vi "CSM - Running Log - DebugTool.vi"() -> ()   [LabVIEW 2017]
doc: "### CSM - Running Log - DebugTool.vi\n\nReal-time tool for viewing the running log of the entire CSM program."
uses:
  _Support/Typedef/_CSM_GlobalLog_MSG.ctl
  _Support/Typedef/_CSM_Response Source Message.ctl
  _Support/Typedef/_CSM_GlobalLog_MSG_TYPE.ctl
  _Support/GlobalEvent/GEvt-Generate with Rule Check.vi
  AdvanceAPI/CSM - Convert Error to Argument.vi
  AdvanceAPI/CSM - Make String Arguments Safe.vi
  AdvanceAPI/CSM - Keywords.vi
  _Support/GlobalEvent/LogFilter/LogFilter - Check.vi
  _Support/GlobalEvent/Cache-GEvt Refs.vi
  _Support/GlobalEvent/LogFilter/LogFilter.lvclass
  Communicable State Machine.lvlib
  addons/Logger/CSM File Logger.lvlib
  _Support/csm-tool-support.lvlib
  _csmHelper/API with lvcsm Support/CSM-Helper API with lvcsm Support.lvlib
panel:
  in  "Check Periodic Messages":bool
  in  "Filter Peroid Logs":bool
  in  "Record.Stop":bool
  in  "Record.Start":bool
  in  "BackTop":bool
  in  "Toolbar.History Length(char)":i32=50000 caption="History(char)" min=1000 max=100000000 step=1
  in  "Clear":bool
  in  "CSM":string(combo)
  in  "Search Button":bool
  in  "Toolbar.Open BD":bool
  in  "Toolbar.Open FP":bool
  out "State History":string
  in  "Tab":enum32{"Error History", "Broadcast Registry"}(tab)
  out "Error History":string
  out "Broadcast Registry":string[][](table)
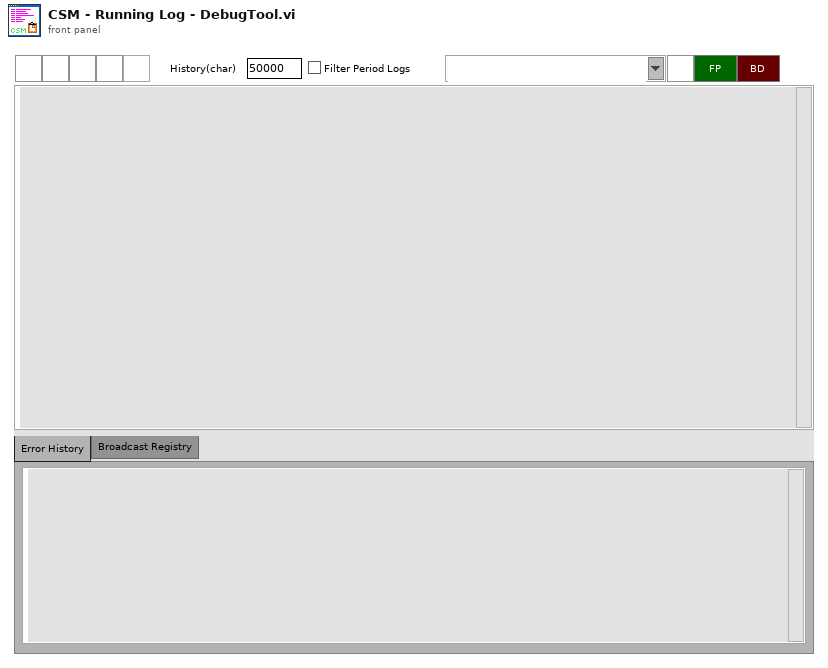
[diagram p1: front panel]
types:
  T1 = cluster{"threashold(#/s)":dbl, "Check Peroid(s)":dbl}
  T2 = typedef "Communicable State Machine.lvlib/_CSM_GlobalLog_MSG.ctl" = cluster{"Name (\"\" to Use UUID)":string, "Current State":string, "Arguments":string, "Source Message":T3, "Source Module":string, "Complete(T)/Start(F)":bool, "LogType":T4, "Time Stamp":timestamp}
  T3 = typedef "Communicable State Machine.lvlib/_CSM_Response Source Message.ctl" = cluster{"‘State":string, "’Arguments":string, "’Error":errorcluster}
  T4 = typedef "Communicable State Machine.lvlib/_CSM_GlobalLog_MSG_TYPE.ctl" = enum16{"User Log", "State Change", "Status", "Interrupt", "Register", "Unregister", "Error Log", "Module Created", "Module Destroyed", "Async Message", "No-Rep Async Message", "Sync Message"}
  T5 = enum32{"Invalid", "Standard", "Closed", "Hidden", "Minimized", "Maximized"}
  T6 = enum32{"invalid app kind", "Development System", "Run Time System", "Student Edition", "Embedded LabVIEW", "Evaluation", "Custom"}
  T7 = typedef "LVPoint32TypeDef.ctl" = cluster{"Horizontal":i32, "Vertical":i32}
  T8 = cluster{"Shift":bool, "Ctrl":bool, "Alt":bool, "Cmd":bool, "Opt":bool}
  T9 = cluster{"Core":cluster{"Current VI Reference":refnum<vi>, "Close Panel on Exit?":bool}, "Toolbar.Advance":refnum<vi>[], "LoggerWatchDogQueue":refnum<queue>, "LogFile":path}
  T10 = cluster{"Current VI Reference":refnum<vi>, "Close Panel on Exit?":bool}
  T11 = typedef "Communicable State Machine.lvlib/CSM - Broadcast Message Type.ctl" = enum16{"<Null>", "Status", "Interrupt"}
  T12 = cluster{string, "Name":string, "Target CSM":string, "Target State":string, "Register Type":T11}[]
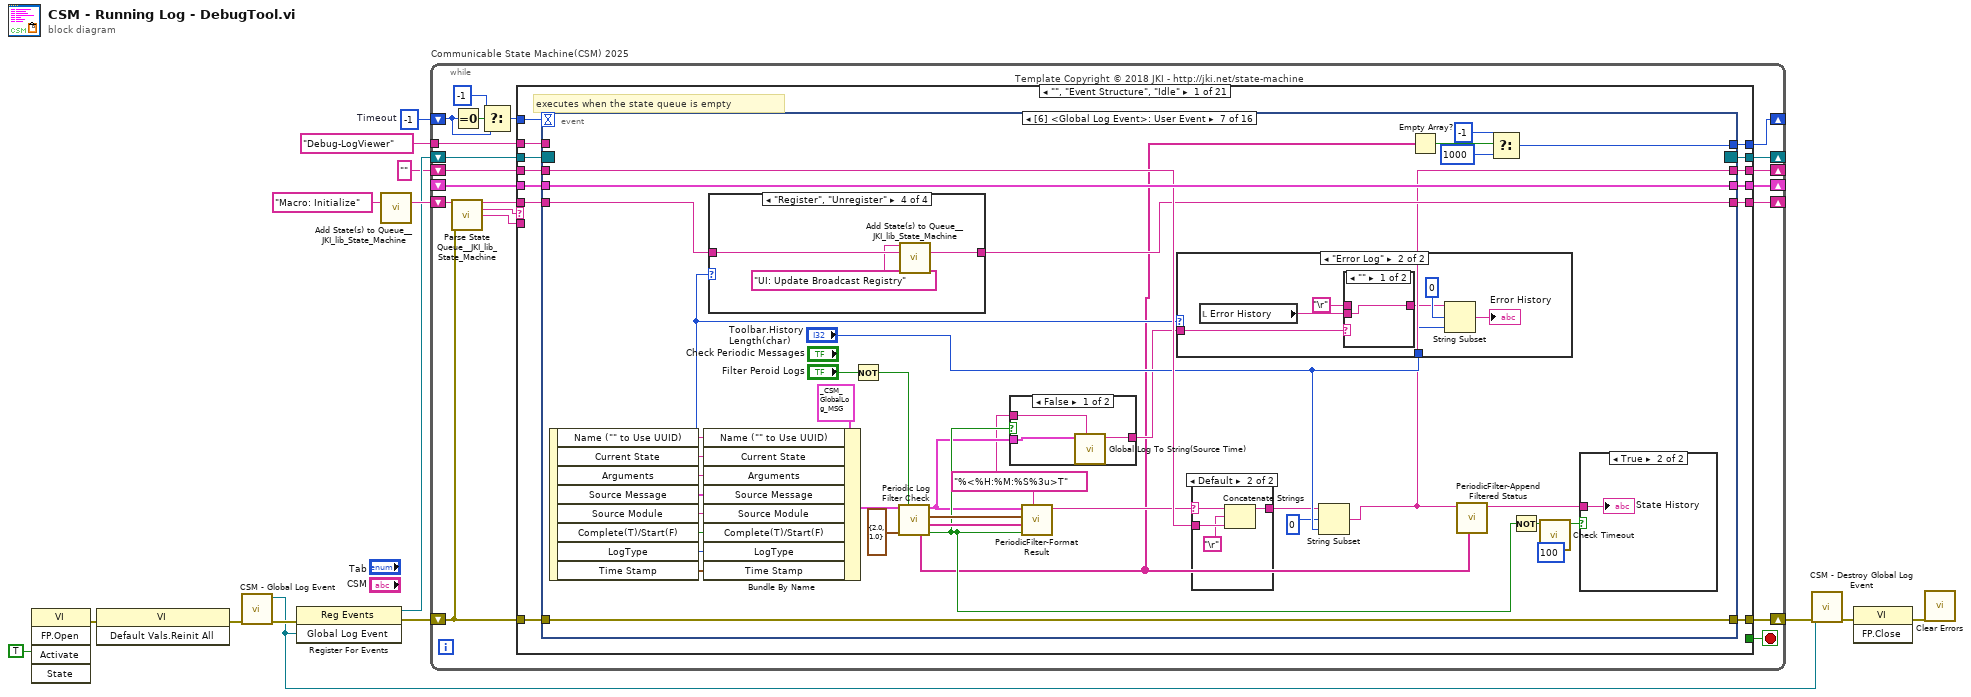
[diagram p0: block diagram]
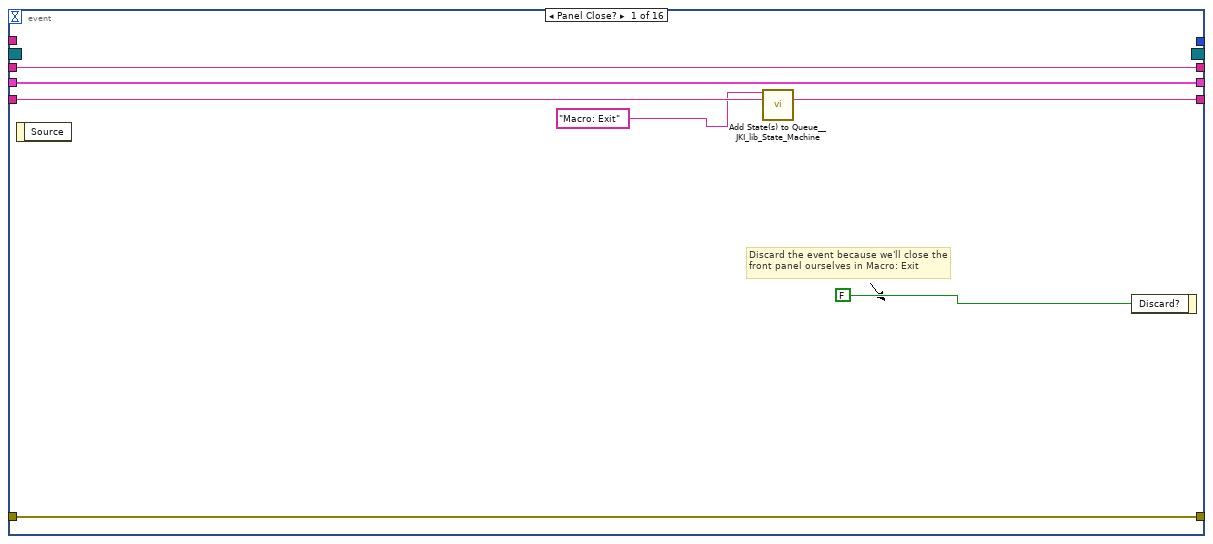
[diagram p2: hidden frame]
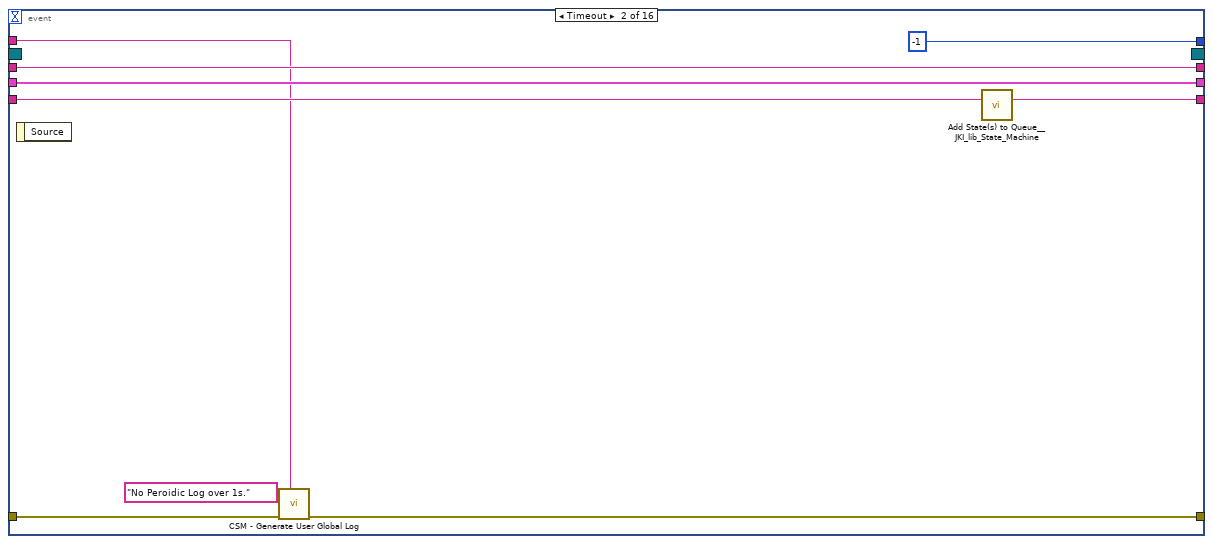
[diagram p3: hidden frame]
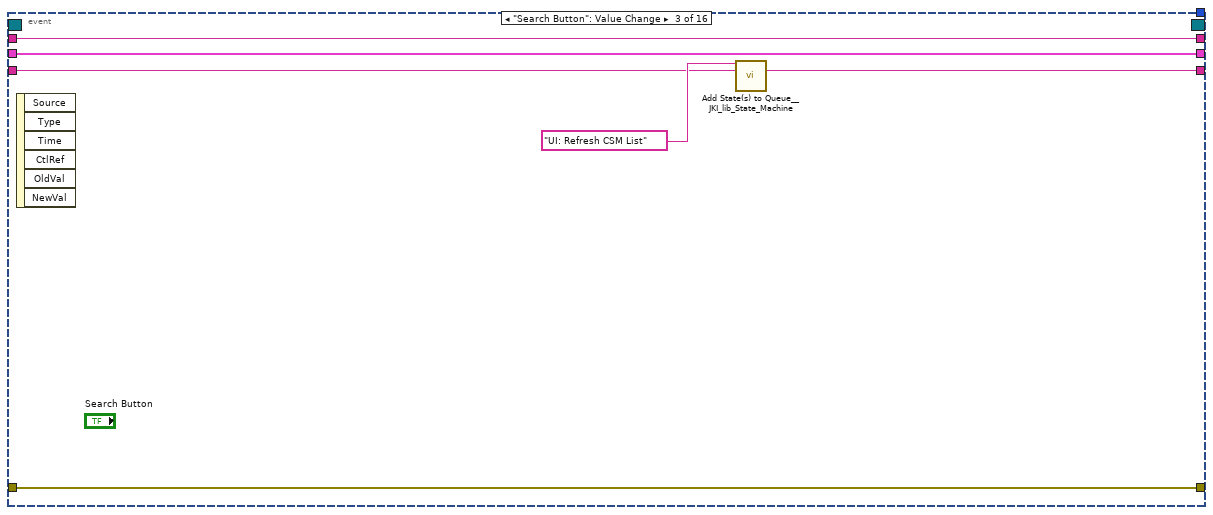
[diagram p4: hidden frame]
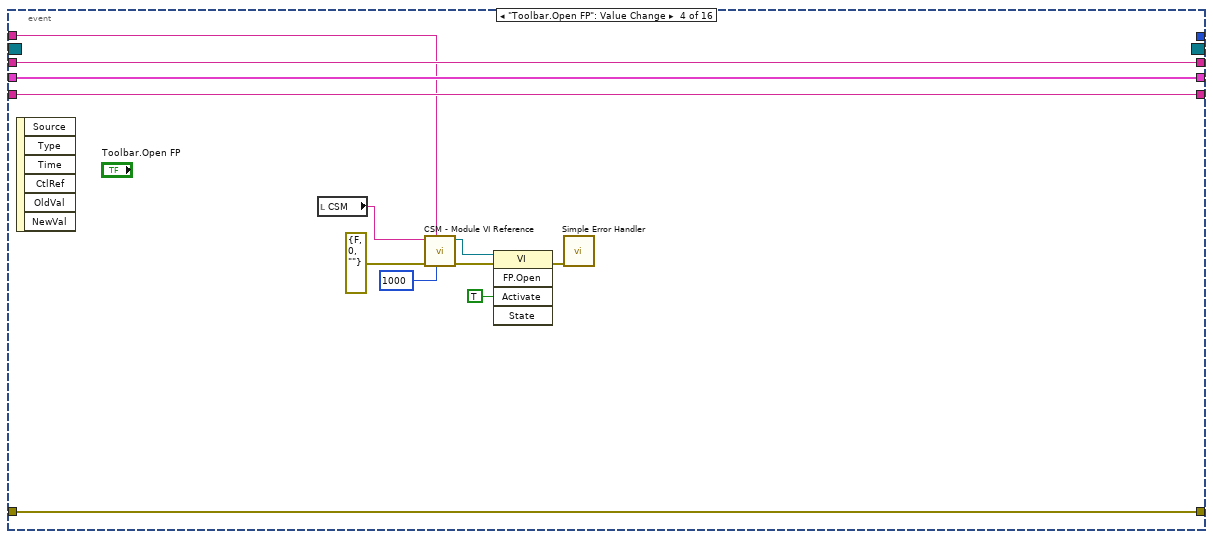
[diagram p5: hidden frame]
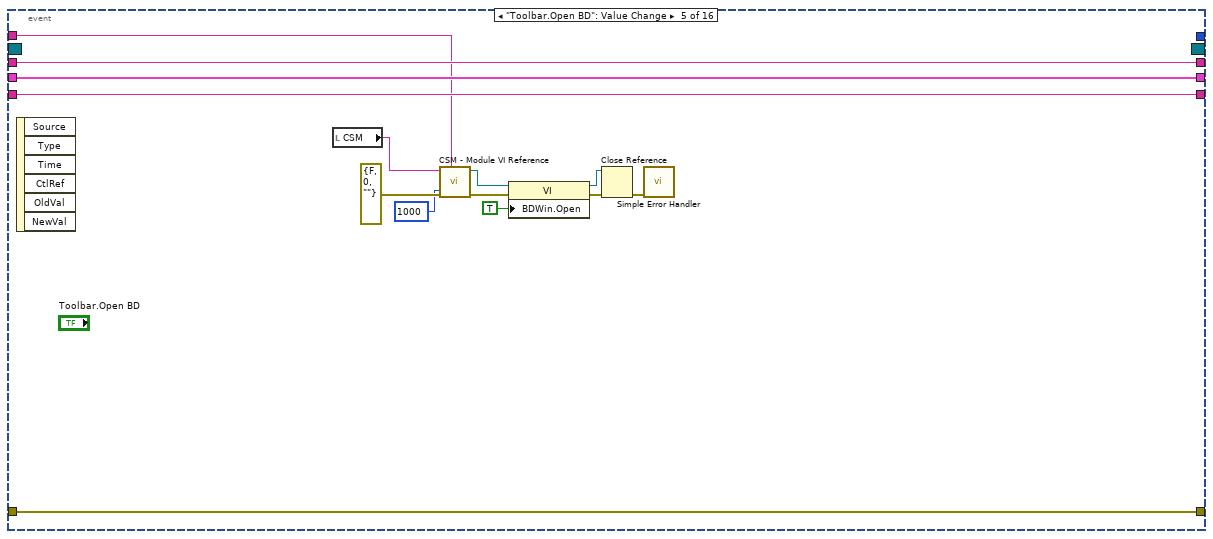
[diagram p6: hidden frame]
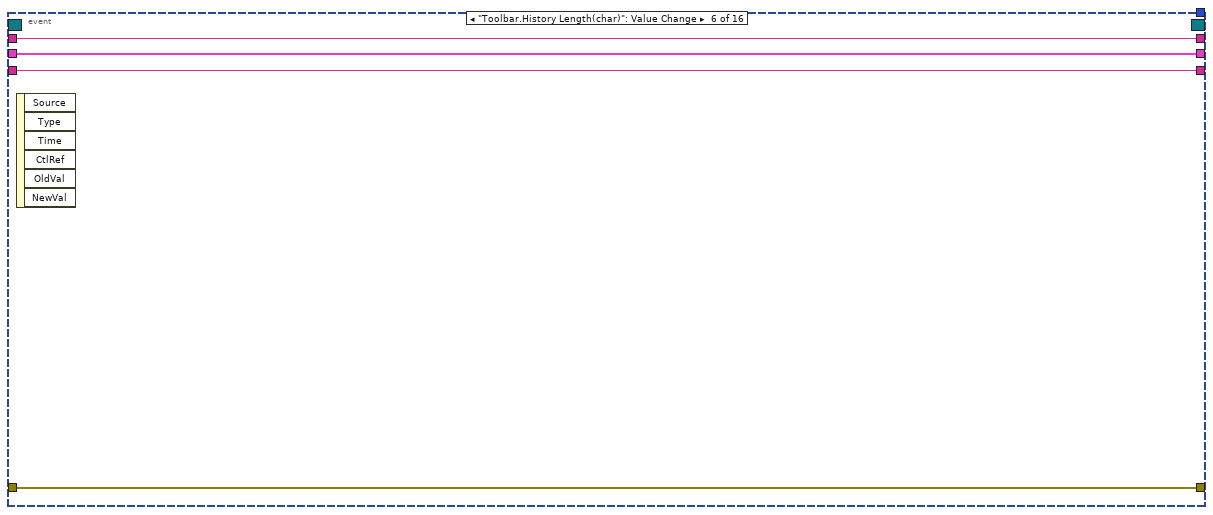
[diagram p7: hidden frame]
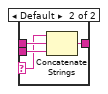
[diagram p12: hidden frame]
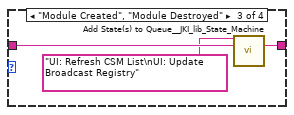
[diagram p15: hidden frame]
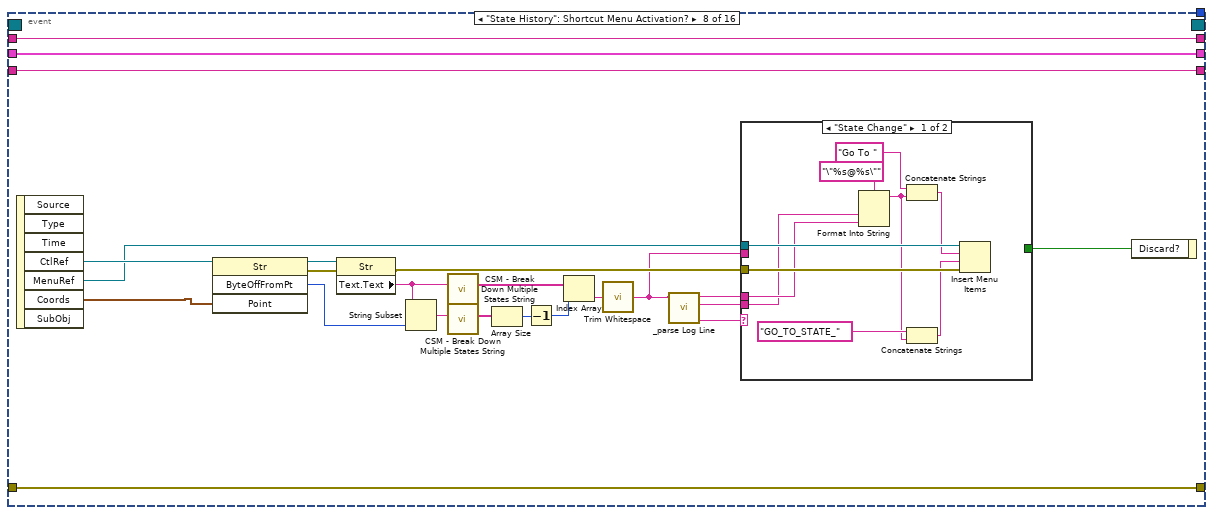
[diagram p16: hidden frame]
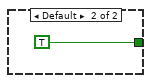
[diagram p17: hidden frame]
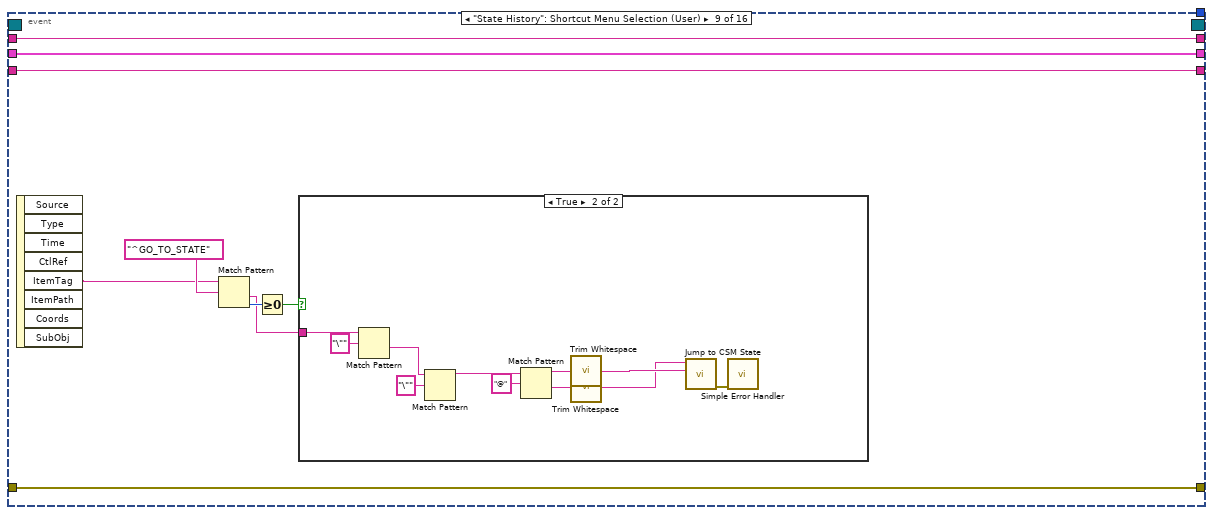
[diagram p18: hidden frame]
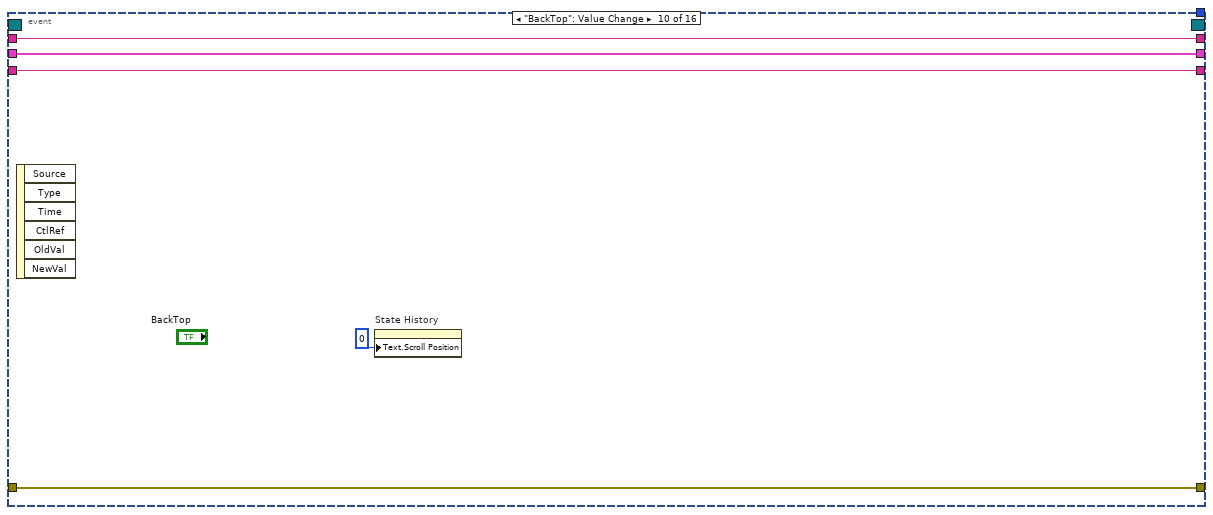
[diagram p20: hidden frame]
diagram:
  w1 = -1  # Timeout
  n1 = invoke class="VI" method="FP.Open"("Activate"=TRUE ("Activate?")) -> (error out=w14:errorcluster)  [unwired: 4 in, 4 out]
  n2 = invoke class="VI" method="Default Vals.Reinit All"(error in=w14) -> (error out=w8:errorcluster)  [unwired: 2 in, 2 out]
  n3 = call "CSM - Global Log Event.vi"("Error In"=w8) -> ("error out"=w12:errorcluster, "Global Log Event"=w11:refnum<user-event>)  [unwired: 9 in]
  n4 = register-events(error in=w12, w11) -> (reference out=w6:refnum<event-registration>, error out=w7:errorcluster)  [unwired: 1 in]
  n5 = call <vilib>:"Add State(s) to Queue__JKI_lib_State_Machine.vi"("State(s) in (\"\")"="Macro: Initialize") -> ("States Out"=w10:string)  [unwired: 14 in]
  n6 = while "Communicable State Machine(CSM) 2025" {
    shift-right: [w28] -> _
    shift-left: _ -> [w27]
    shift-right: [w31] -> w5
    shift-left: w7 -> [w26]
    shift-right: [w30] -> _
    shift-left: w10 -> [w32]
    shift-right: [w24] -> _
    shift-left: w6 -> [w25]
    tunnel: "Debug-LogViewer" ("Current Module(\"\" to generate an ID)") -> [w23]
    shift-right: [w21] -> _
    shift-left: "" ("String Cache") -> [w22]
    shift-right: [w20] -> _
    shift-left: w1 -> [w17]
    stop <- w29 stop-if-true
    # "Template Copyright © 2018 JKI - http://jki.net/state-machine"
    n7 = call <vilib>:"Parse State Queue__JKI_lib_State_Machine.vi"("State Queue"=w32, "Error In (no error)"=w26) -> ("Remaining States"=w34:string, "Current State"=w35:string, "Arguments"=w33:string)  [unwired: 11 in]
    n8 = Equal To 0?(x=w17) -> (x = 0?=w19:bool)
    n9 = Select(t=-1 ("Timeout"), s=w19, f=w17) -> (s? t:f=w18:i32)
    n10 = case shown="\"\", \"Event Structure\", \"Idle\"" w35 {
      selector: w35 -> [_ _ w296 _ _ _ _ _ _ _ _ _ _ _ _ _ _ _ _ _ _]
      tunnel: w34 -> [w48 w292 w300 w322 w331 w339 w346 w357 w367 w376 w383 w392 w404 w418 w495 w503 w532 w556 w564 w572 w585]
      tunnel: w33 -> [_ _ _ _ _ _ _ _ _ _ _ _ w399 w412 _ _ _ _ _ _ _]
      tunnel: w27 -> [w46 w289 w298 w315 w328 w337 w343 _ w366 w371 w380 w387 w402 w414 w494 w502 w527 w555 w561 w569 w582]
      tunnel: [w45 w290 w302 w319 errorcluster {"status"=FALSE, "code"=0, "source"=""} ("error out") w336 w344 w354 w359 w372 w381 w390 w400 w415 w496 w504 w533 w557 w562 w570 w583] -> w31
      tunnel: w26 -> [w44 w290 w301 w319 w327 w336 w344 w354 w359 w373 w381 w390 w401 w416 w496 w504 w533 w557 w562 w570 w583]
      tunnel: [w47 w291 w299 w321 w330 w338 w345 w356 w367 w375 w382 w391 w403 w417 w495 w503 w532 w556 w563 w571 w584] -> w30
      tunnel: [_ _ _ _ _ TRUE _ _ _ _ _ _ _ _ _ _ _ _ _ _ _] -> w29
      tunnel: [w43 w289 w298 w320 w328 w337 w343 w355 w363 w371 w380 w387 w402 w414 w494 w502 w527 w555 w561 w569 w582] -> w28
      tunnel: w18 -> [w42 w286 w293 w307 w323 w332 w340 w347 w358 w368 w377 w384 w396 w409 w484 w497 w513 w540 w558 w565 w573]
      tunnel: w25 -> [w41 w288 w295 w309 w325 w334 w342 w352 w365 w370 w379 w389 w398 w411 w493 w501 w531 w554 w560 w567 w575]
      tunnel: [w40 w288 w295 w309 w325 w334 w342 w352 w365 w370 w379 w389 w398 w411 w493 w501 w531 w554 w560 w567 w575] -> w24
      tunnel: w23 -> [w39 _ _ _ _ _ _ _ _ _ _ _ _ _ _ _ _ _ _ _ _]
      tunnel: w22 -> [w38 w287 w294 w308 w324 w333 w341 w351 w364 w369 w378 w388 w397 w410 w492 w500 w530 w553 w559 w566 w574]
      tunnel: [w37 w287 w294 w308 w324 w333 w341 w351 w364 w369 w378 w388 w397 w410 w492 w500 w530 w553 w559 w566 w574] -> w21
      tunnel: [w36 w286 w293 w307 w323 w332 w340 w347 w358 w368 w377 w384 w396 w409 w484 w497 w513 w540 w558 w565 w573] -> w20
      frame "", "Event Structure", "Idle" {
        # "executes when the state queue is empty"
        n11 = event shown="[6] <Global Log Event>: User Event" {
          selector: w41 -> [_ _ _ _ _ _ _ _ _ _ _ _ _ _ _ _]
          dyn-events: [_ _ _ _ _ _ _ _ _ _ _ _ _ _ _ _] -> w40
          timeout: w42 -> [_ _ _ _ _ _ _ _ _ _ _ _ _ _ _ _]
          tunnel: w48 -> [w55 w64 w66 w81 w96 w100 w128 w190 w210 w226 w239 w246 w248 w265 w275 w281]
          tunnel: [w54 w63 w65 w81 w96 w100 w127 w190 w210 w226 w239 w246 w247 w264 w276 w282] -> w47
          tunnel: w46 -> [w52 w61 w70 w82 w94 w98 w137 w188 w208 w224 w229 w244 w257 w271 w278 w284]
          tunnel: [w53 w58 w69 w80 w95 w99 w138 w189 w209 w225 w238 w245 w259 w273 w279 w285] -> w45
          tunnel: w44 -> [w53 w62 w69 w80 w95 w99 w138 w189 w209 w225 w238 w245 _ w273 w279 w285]
          tunnel: [w52 w61 w70 w82 w94 w98 w137 w188 w208 w224 w229 w244 w260 w267 w278 w284] -> w43
          tunnel: w39 -> [_ w57 _ w77 w91 _ _ _ _ _ _ _ _ _ _ _]
          tunnel: w38 -> [w49 w60 w68 w79 w93 w97 w129 w187 w207 w223 w237 _ w262 w272 w277 w283]
          tunnel: [w49 w60 w68 w79 w93 w97 w103 w187 w207 w223 w237 w243 w262 w272 w277 w283] -> w37
          tunnel: [_ -1 ("Timeout") _ _ _ _ w121 _ _ _ _ _ _ _ _ _] -> w36
          event Panel Close? {
            # "Discard the event because we'll close the front panel ourselves in Macro: Exit"
            n12 = event-data() -> ()  [unwired: 1 in, 1 out]
            n13 = call <vilib>:"Add State(s) to Queue__JKI_lib_State_Machine.vi"("State(s) in Front (\"\")"="Macro: Exit", "State(s) in (\"\")"=w55) -> ("States Out"=w54:string)  [unwired: 13 in]
            n14 = event-data("Discard?"=FALSE) -> ()  [unwired: 1 in, 1 out]
          }
          event Timeout {
            n15 = event-data() -> ()  [unwired: 1 in, 1 out]
            n16 = call "CSM - Generate User Global Log.vi"("Place (\"\" to Use VI's Name)"=w57, "Error In"=w62, "Log"="No Peroidic Log over 1s.") -> ("error out"=w58:errorcluster)  [unwired: 8 in]
            n17 = call <vilib>:"Add State(s) to Queue__JKI_lib_State_Machine.vi"("State(s) in (\"\")"=w64) -> ("States Out"=w63:string)  [unwired: 14 in]
          }
          event "Search Button": Value Change {
            n18 = event-data() -> ()  [unwired: 1 in, 6 out]
            n19 = call <vilib>:"Add State(s) to Queue__JKI_lib_State_Machine.vi"("State(s) in Front (\"\")"="UI: Refresh CSM List" ("State(s) in Front (\"\")"), "State(s) in (\"\")"=w66) -> ("States Out"=w65:string)  [unwired: 13 in]
          }
          event "Toolbar.Open FP": Value Change {
            n20 = event-data() -> ()  [unwired: 1 in, 6 out]
            n21 = local read "CSM"() -> (w76:string)
            n22 = call "CSM - Module VI Reference.vi"("Response Timeout (-2 Using Global Settings)"=1000 ("Response Timeout(5000 ms)"), "Current Module (\"\" to Generate an ID)"=w77, "error in (no error)"=errorcluster {"status"=FALSE, "code"=0, "source"=""}, "CSM Name"=w76) -> ("error out"=w72:errorcluster, "CSM Module VIRef"=w73:refnum<vi>)  [unwired: 6 in]
            n23 = invoke on="Invoke Node" class="VI" method="FP.Open"(reference=w73, error in=w72, "Activate"=TRUE ("Activate?")) -> (error out=w78:errorcluster)  [unwired: 2 in, 4 out]
            n24 = call <vilib>:"Simple Error Handler.vi"("error in (no error)"=w78) -> ()  [unwired: 4 in, 5 out]
          }
          event "Toolbar.Open BD": Value Change {
            n25 = event-data() -> ()  [unwired: 1 in, 6 out]
            n26 = local read "CSM"() -> (w90:string)
            n27 = call "CSM - Module VI Reference.vi"("Response Timeout (-2 Using Global Settings)"=1000 ("Response Timeout(5000 ms)"), "Current Module (\"\" to Generate an ID)"=w91, "error in (no error)"=errorcluster {"status"=FALSE, "code"=0, "source"=""}, "CSM Name"=w90) -> ("error out"=w83:errorcluster, "CSM Module VIRef"=w88:refnum<vi>)  [unwired: 6 in]
            n28 = property class="VI"(reference=w88, error in=w83, "BDWin.Open"=TRUE ("Block Diagram Window:Open")) -> (reference out=w86:refnum<vi>, error out=w85:errorcluster)
            n29 = Close Reference(reference=w86, error in (no error)=w85) -> (error out=w92:errorcluster)
            n30 = call <vilib>:"Simple Error Handler.vi"("error in (no error)"=w92) -> ()  [unwired: 4 in, 5 out]
          }
          event "Toolbar.History Length(char)": Value Change {
            n31 = event-data() -> ()  [unwired: 1 in, 6 out]
          }
          event User Event {
            w104 = "%<%H:%M:%S%3u>T" ("Time format string")
            n32 = event-data() -> ("Name (\"\" to Use UUID)"=w135:string, "Current State"=w134:string, "Arguments"=w133:string, "Source Message"=w132:T3, "Source Module"=w131:string, "Complete(T)/Start(F)"=w130:bool, "LogType"=w126:T4, "Time Stamp"=w113:timestamp)  [unwired: 1 in]
            n33 = Bundle By Name(cluster=T2 {"Name (\"\" to Use UUID)"="", "Current State"="", "Arguments"="", "Source Message"={"‘State"="", "’Arguments"="", "’Error"={"status"=FALSE, "code"=0, "source"=""}}, "Source Module"="", "Complete(T)/Start(F)"=FALSE, "LogType"=enum."State Change", "Time Stamp"=timestamp(0 s since 1904-01-01)} ("Cross CSM Data"), "Name (\"\" to Use UUID)"=w135, "Current State"=w134, "Arguments"=w133, "Source Message"=w132, "Source Module"=w131, "Complete(T)/Start(F)"=w130, "LogType"=w126, "Time Stamp"=w113) -> (w124:T2)
            n34 = case shown="\"Register\", \"Unregister\"" w126 {
              tunnel: w128 -> [w160 w161 w164 w167]
              tunnel: [w160 w161 w163 w166] -> w127
              frame "State Change", Default {
              }
              frame "User Log" {
              }
              frame "Module Created", "Module Destroyed" {
                n35 = call <vilib>:"Add State(s) to Queue__JKI_lib_State_Machine.vi"("State(s) in Front (\"\")"="UI: Refresh CSM List\nUI: Update Broadcast Registry" ("State(s) in Front (\"\")"), "State(s) in (\"\")"=w164) -> ("States Out"=w163:string)  [unwired: 13 in]
              }
              frame "Register", "Unregister" {
                n36 = call <vilib>:"Add State(s) to Queue__JKI_lib_State_Machine.vi"("State(s) in Front (\"\")"="UI: Update Broadcast Registry" ("State(s) in Front (\"\")"), "State(s) in (\"\")"=w167) -> ("States Out"=w166:string)  [unwired: 13 in]
              }
            }
            n37 = Not(x="Filter Peroid Logs") -> (.not. x?=w122:bool)
            n38 = call "Periodic Log Filter Check.vi"("Cross CSM Data"=w124, "Reset?"=w122, "Settings"=T1 {"threashold(#/s)"=2.0, "Check Peroid(s)"=1.0}) -> ("Cross CSM Data Out"=w106:T2, "Current Time"=w112:timestamp, "Additional Info"=w111:string[], "Filtered Status"=w101:string[], "Filtered"=w109:bool)  [unwired: 8 in]
            n39 = case shown="False" w109 {
              tunnel: w106 -> [w146 _]
              tunnel: [w145 _] -> w105
              tunnel: w104 -> [w144 _]
              frame False {
                n40 = call "Global Log To String(Source Time).vi"("Format String"=w144, "Log"=w146) -> ("Log String"=w145:string)  [unwired: 8 in]
              }
              frame True {
              }
            }
            n41 = call "PeriodicFilter-Format Result.vi"("Time Format String"=w104, "Filtered"=w109, "Additional Info"=w111, "Current Time"=w112, "Cross CSM Data In"=w106) -> ("States"=w110:string)  [unwired: 6 in]
            n42 = case shown="\"Error Log\"" w126 {
              tunnel: "Toolbar.History Length(char)" -> [_ w149]
              tunnel: w105 -> [_ w148]
              frame "User Log", Default {
              }
              frame "Error Log" {
                n43 = local read "Error History"() -> (w153:string)
                n44 = case shown="\"\"" w148 {
                  selector: w148 -> [_ w156]
                  tunnel: "\r" -> [_ w159]
                  tunnel: w153 -> [w155 w158]
                  tunnel: [w155 w157] -> w151
                  frame "" {
                  }
                  frame Default {
                    n45 = Concatenate Strings(w156, w159, w158) -> (w157:string)
                  }
                }
                n46 = String Subset(string=w151, offset (0)=0, length (rest)=w149) -> (substring=→"Error History":string)
              }
            }
            n47 = case shown="Default" w110 {
              selector: w110 -> [_ w142]
              tunnel: w129 -> [w139 w143]
              tunnel: [w139 w141] -> w107
              frame "" {
              }
              frame Default {
                n48 = Concatenate Strings(w142, "\r", w143) -> (w141:string)
              }
            }
            n49 = String Subset(string=w107, offset (0)=0, length (rest)="Toolbar.History Length(char)") -> (substring=w103:string)
            n50 = Empty Array?(array=w101) -> (empty?=w118:bool)
            n51 = call "PeriodicFilter-Append Filtered Status.vi"("Filtered Status"=w101, "String Cache In"=w103) -> ("String Cache Out"=w102:string)  [unwired: 9 in]
            n52 = Select(t=-1 ("Timeout"), s=w118, f=1000 ("Timeout")) -> (s? t:f=w121:i32)
            n53 = Not(x=w109) -> (.not. x?=w115:bool)
            n54 = call "Check Timeout.vi"("Timeout Expected (ms)"=100 ("Timeout Expected(ms)"), "Force Timeout?"=w115) -> ("Timeout"=w116:bool)  [unwired: 6 in]
            n55 = case shown="True" w116 {
              tunnel: w102 -> [_ w147]
              frame False {
              }
              frame True {
                "State History" <- w147
              }
            }
          }
          event "State History": Shortcut Menu Activation? {
            n56 = event-data() -> ("CtlRef"=w170:refnum<vi>, "MenuRef"=w169:refnum<k9>, "Coords"=w168:T7)  [unwired: 1 in, 4 out]
            n57 = invoke class="Str" method="ByteOffFromPt"(reference=w170, "Point"=w168) -> (reference out=w186:refnum<vi>, error out=w184:errorcluster, "ByteOffFromPt"=w185:i32)  [unwired: 2 in, 1 out]
            n58 = property class="Str"(reference=w186, error in=w184) -> (error out=w176:errorcluster, "Text.Text"=w182:string)  [unwired: 1 out]
            n59 = String Subset(string=w182, length (rest)=w185) -> (substring=w183:string)  [unwired: 1 in]
            n60 = call "CSM - Break Down Multiple States String.vi"("States"=w182) -> ("Multiple States"=w181:string[])  [unwired: 10 in]
            n61 = call "CSM - Break Down Multiple States String.vi"("States"=w183) -> ("Multiple States"=w180:string[])  [unwired: 10 in]
            n62 = Array Size(array=w180) -> (size(s)=w179:i32)
            n63 = Decrement(x=w179) -> (x-1=w178:i32)
            n64 = Index Array(array=w181, index=w178) -> (element=w177:string)
            n65 = call <vilib>:"Trim Whitespace.vi"("string"=w177) -> ("trimmed string"=w175:string)  [unwired: 1 in]
            n66 = call "_parse Log Line.vi"("String"=w175) -> ("LogType"=w174:string, "State"=w172:string, "CSM"=w173:string)  [unwired: 8 in]
            n67 = case shown="\"State Change\"" w174 {
              tunnel: w169 -> [w200 _]
              tunnel: w175 -> [_ _]
              tunnel: w176 -> [w198 _]
              tunnel: [_ TRUE] -> w171
              tunnel: w173 -> [w196 _]
              tunnel: w172 -> [w195 _]
              frame "State Change" {
                n68 = Format Into String(format string="\"%s@%s\"", w195, w196) -> (resulting string=w191:string)  [unwired: 2 in, 1 out]
                n69 = Concatenate Strings("Go To " ("format string"), w191) -> (w194:string)
                n70 = Concatenate Strings("GO_TO_STATE_" ("item tags"), w191) -> (w192:string)
                n71 = Insert Menu Items(6:w198, 7:w192, 8:w194, 9:w200) -> ()  [unwired: 2 in, 3 out]
              }
              frame Default {
              }
            }
            n72 = event-data("Discard?"=w171) -> ()  [unwired: 1 in, 1 out]
          }
          event "State History": Shortcut Menu Selection (User) {
            n73 = event-data() -> ("ItemTag"=w202:string)  [unwired: 1 in, 7 out]
            n74 = Match Pattern(string=w202, regular expression="^GO_TO_STATE") -> (after substring=w203:string, offset past match=w205:i32)  [unwired: 1 in, 2 out]
            n75 = Greater Or Equal To 0?(x=w205) -> (x >= 0?=w204:bool)
            n76 = case shown="True" w204 {
              tunnel: w203 -> [_ w221]
              frame False {
              }
              frame True {
                n77 = Match Pattern(string=w221, regular expression="\"") -> (after substring=w218:string)  [unwired: 1 in, 3 out]
                n78 = Match Pattern(string=w218, regular expression="\"") -> (before substring=w217:string)  [unwired: 1 in, 3 out]
                n79 = Match Pattern(string=w217, regular expression="@") -> (before substring=w215:string, after substring=w214:string)  [unwired: 1 in, 2 out]
                n80 = call <vilib>:"Trim Whitespace.vi"("string"=w215) -> ("trimmed string"=w213:string)  [unwired: 1 in]
                n81 = call <vilib>:"Trim Whitespace.vi"("string"=w214) -> ("trimmed string"=w212:string)  [unwired: 1 in]
                n82 = call "Jump to CSM State.vi"("State"=w213, "Name"=w212) -> ("error out"=w211:errorcluster)  [unwired: 9 in]
                n83 = call <vilib>:"Simple Error Handler.vi"("error in (no error)"=w211) -> ()  [unwired: 4 in, 5 out]
              }
            }
          }
          event "BackTop": Value Change {
            n84 = event-data() -> ()  [unwired: 1 in, 6 out]
            n85 = property on="State History" class="Str"("Text.Scroll Position"=u32 0) -> ()  [unwired: 2 in, 2 out]
          }
          event Key Down {
            n86 = event-data() -> ("Char"=w227:i16, "PlatMods"=w232:T8)  [unwired: 1 in, 8 out]
            n87 = Unbundle By Name(w232) -> ("Ctrl"=w231:bool)
            n88 = String To Byte Array(string="Qq") -> (unsigned byte array=w234:u8[])
            n89 = Search 1D Array(1D array=w234, element=w227) -> (index of element=w235:i32)  [unwired: 1 in]
            n90 = Unbundle By Name(w229) -> ("Toolbar.Advance"=w228:refnum<vi>[])
            n91 = Greater Or Equal To 0?(x=w235) -> (x >= 0?=w236:bool)
            n92 = And(x=w236, y=w231) -> (x .and. y?=w230:bool)
            n93 = case shown="True" w230 {
              tunnel: w228 -> [_ w240]
              frame False {
              }
              frame True {
                n94 = for {
                  tunnel: w240 -> [w242] mode=indexing
                  n95 = property class="Bool"(reference=w242, "Visible"=TRUE) -> ()  [unwired: 1 in, 2 out]
                }
              }
            }
          }
          event "Clear": Value Change {
            w243 = "" ("String Cache")
            n96 = event-data() -> ()  [unwired: 1 in, 6 out]
            n97 = local write "State History"(w243) -> ()
            n98 = local write "Error History"(w243) -> ()
          }
          event "Record.Start": Value Change {
            n99 = event-data() -> ()  [unwired: 1 in, 1 out]
            n100 = Unbundle By Name(w257) -> ("Core.Current VI Reference"=w256:refnum<vi>)
            n101 = property class="VI"(reference=w256) -> (error out=w255:errorcluster, "OwningApp"=w254:refnum<vi>)  [unwired: 1 in, 1 out]
            n102 = property class="App"(reference=w254, error in=w255) -> (error out=w252:errorcluster, "Project.ActiveProject"=w253:refnum<vi>)  [unwired: 1 out]
            n103 = property class="Project"(reference=w253, error in=w252) -> ("Name"=w251:string)  [unwired: 2 out]
            n104 = String To Path(string=w251) -> (path=w250:path)
            n105 = call "CSM - Start File Logger.vi"("Log File Path"=w250) -> ("error out"=w259:errorcluster, "Log File"=w258:path, "Watchdog Queue"=w261:refnum<queue>)  [unwired: 8 in]
            n106 = Bundle By Name(cluster=w257, "LoggerWatchDogQueue"=w261, "LogFile"=w258) -> (w260:T9)
            n107 = call <vilib>:"Add State(s) to Queue__JKI_lib_State_Machine.vi"("State(s) in Front (\"\")"="UI: Update Toolbar" ("State(s) in Front (\"\")"), "State(s) in (\"\")"=w248) -> ("States Out"=w247:string)  [unwired: 13 in]
          }
          event "Record.Stop": Value Change {
            n108 = event-data() -> ()  [unwired: 1 in, 6 out]
            n109 = Unbundle By Name(w271) -> ("LoggerWatchDogQueue"=w270:refnum<queue>)
            n110 = Release Queue(queue=w270, force destroy? (F)=TRUE) -> (error out=w268:errorcluster)  [unwired: 1 in, 2 out]
            n111 = call <vilib>:"Clear Errors.vi"("error in (no error)"=w268) -> ()  [unwired: 5 in, 2 out]
            n112 = Bundle By Name(cluster=w271, "LogFile"=path "") -> (w267:T9)
            n113 = call <vilib>:"Add State(s) to Queue__JKI_lib_State_Machine.vi"("State(s) in Front (\"\")"="UI: Update Toolbar" ("State(s) in Front (\"\")"), "State(s) in (\"\")"=w265) -> ("States Out"=w264:string)  [unwired: 13 in]
          }
          event Pane Size {
            n114 = event-data() -> ()  [unwired: 1 in, 6 out]
            n115 = call <vilib>:"Add State(s) to Queue__JKI_lib_State_Machine.vi"("State(s) in (\"\")"=w275, "State(s) at Back (\"\")"="UI: Resize Tab Content" ("State(s) in Front (\"\")")) -> ("States Out"=w276:string)  [unwired: 13 in]
          }
          event "Tab": Value Change {
            n116 = event-data() -> ()  [unwired: 1 in, 6 out]
            n117 = call <vilib>:"Add State(s) to Queue__JKI_lib_State_Machine.vi"("State(s) in Front (\"\")"="UI: Update Broadcast Registry" ("State(s) in Front (\"\")"), "State(s) in (\"\")"=w281) -> ("States Out"=w282:string)  [unwired: 13 in]
          }
        }
      }
      frame "---------- Core ----------" {
        # "Do not put any code in this frame.\n(it is a separator no-op)"
        n118 = call <vilib>:"Add State(s) to Queue__JKI_lib_State_Machine.vi"("State(s) in (\"\")"=w292) -> ("States Out"=w291:string)  [unwired: 14 in]
      }
      frame Default {
        w305 = 42 items=["No error", "Argument error", "Memory is full", "Out of zone", "End of file", "File already open", "Generic file I/O error", "File not found", "File permission error", "Disk is full", "Duplicate path", "Too many files open", "System feature not enabled", "Resource file not found", "Cannot add resource", "Resource not found", "Image not found", "Image memory error", "Pen does not exist", "Config type invalid", "Config token not found", "Config parse error", "Config memory error", "Bad external code format", "Bad external code offset", "External code not present", "Null window", "Destroy window error", "Null menu", "Print aborted", "Bad print record", "Print driver error", "Windows error during printing", "Memory error during printing", "Print dialog error", "Generic print error", "Invalid device refnum", "Device not found", "Device parameter error", "Device unit error", "Cannot open device", "Device call aborted", "Generic error", "Cancelled by user", "Object ID too low", "Object ID too high", "Object not in heap", "Unknown heap", "Unknown object (invalid DefProc)", "Unknown object (DefProc not in table)", "Message out of range", "Invalid (null) method", "Unknown message", "Manager call not supported", "Bad address", "Network operation in progress", "Network operation timed out", "Connection is busy", "Network attribute not supported", "Network error", "Address in use", "System out of memory", "Connection aborted", "Connection refused", "Not connected", "Already connected", "Connection closed", "Initialization error (interapplication manager)", "Bad occurrence", "Wait on unbound occurrence handler", "Occurrence queue overflow", "Datalog type conflict", "Unused", "Unrecognized type (interapplication manager)", "Memory corrupt", "Failed to make temporary DLL", "Old CIN version", "Drag socket not found", "Failed to load drop-object", "Failed to register OLE object", "Failed to release OLE object", "Format specifier type mismatch", "Unknown format specifier", "Too few format specifiers", "Too many format specifiers", "Scan failed", "Newer CIN version", "Error converting to variant", "Runtime menu error", "Password tampered", "Variant attribute not found", "Incompatible variant data type", "Event data is not available", "Event Store is not present", "Occurrence is not found", "Event Queue is not created", "Event info is not available", "Refnum passed is NULL", "Error retrieving Class GUID", "Error retrieving CoClass GUID", "Error retrieving TypeLib GUID.", "Bad built application magic bytes.", "Specific driver is different from the specific driver associated with the Logical Name.", "There is no session opened to the class driver.", "Max Error", "MAX - Error with config objects", "MAX - Error loading configuration", "MAX - Group not supported"]
        # "Current State"
        # "Do not delete, rename, or modify this frame.\n(this is used to capture unhandled states and typos)"
        # "Handle mistyped state name (developer tool)"
        n119 = Format Into String(format string="Software Exception: Unhandled State \"%s\"." ("message"), error in=w301, w296) -> (resulting string=w304:string, error out=w303:errorcluster)  [unwired: 1 in]
        n120 = call <vilib>:"Error Cluster From Error Code.vi"("show call chain? (False)"=TRUE, "error in (no error)"=w303, "error message (\"\")"=w304, "error code (0)"=w305) -> ("error out"=w302:errorcluster)  [unwired: 5 in]
        n121 = call <vilib>:"Add State(s) to Queue__JKI_lib_State_Machine.vi"("State(s) in (\"\")"=w300) -> ("States Out"=w299:string)  [unwired: 14 in]
      }
      frame "Initialize Core Data" {
        # "Do not delete, rename, or modify this frame.\n(this is used to determine panel behavior on exit)"
        # "originally closed?"
        # "exe?"
        # "If panel starts closed or is an EXE, then close it when we exit"
        n122 = property class="VI"() -> ("FP.State"=w312:T5)  [unwired: 2 in, 2 out]
        n123 = property class="App"() -> ("App.Kind"=w318:T6)  [unwired: 2 in, 2 out]
        n124 = control-ref of="Current VI Reference"() -> (w313:refnum<vi>)
        n125 = Equal?(x=w312, y=T5."Closed" ("Front Panel Window:State")) -> (x = y?=w310:bool)
        n126 = Equal?(x=w318, y=T6."Run Time System" ("Application:Kind")) -> (x = y?=w316:bool)
        n127 = Or(x=w310, y=w316) -> (x .or. y?=w314:bool)
        n128 = Bundle By Name(cluster=w315, "Core.Current VI Reference"=w313, "Core.Close Panel on Exit?"=w314) -> (w320:T9)
        n129 = call <vilib>:"Add State(s) to Queue__JKI_lib_State_Machine.vi"("State(s) in (\"\")"=w322) -> ("States Out"=w321:string)  [unwired: 14 in]
      }
      frame "Error Handler" {
        # "Unhandled Error -- Display it"
        # "Handle any errors here.\nYou can also output any states to clean-up after errors occur"
        # "Clear error"
        n130 = call <vilib>:"General Error Handler.vi"("error in (no error)"=w327) -> ()  [unwired: 10 in, 5 out]
        n131 = call <vilib>:"Add State(s) to Queue__JKI_lib_State_Machine.vi"("State(s) in Front (\"\")"="/* Post Error States", "State(s) in (\"\")"=w331) -> ("States Out"=w330:string)  [unwired: 13 in]
      }
      frame "Exit" {
        # "Do not put any code in this frame.\n(No errors that occur here will be handled.)"
        n132 = call <vilib>:"Add State(s) to Queue__JKI_lib_State_Machine.vi"("State(s) in (\"\")"=w339) -> ("States Out"=w338:string)  [unwired: 14 in]
      }
      frame "---------- Data ----------" {
        # "Do not put any code in this frame.\n(It is a separator no-op. You can make a copy of this frame to create a new Data frame)"
        n133 = call <vilib>:"Add State(s) to Queue__JKI_lib_State_Machine.vi"("State(s) in (\"\")"=w346) -> ("States Out"=w345:string)  [unwired: 14 in]
      }
      frame "Data: Initialize" {
        w348 = refnum<queue> refnum  # LoggerWatchDogQueue
        w349 = path ""  # LogFile
        w350 = refnum<vi>[] []  # Toolbar.Advance
        w353 = T10 {"Current VI Reference"=refnum, "Close Panel on Exit?"=FALSE}  # Core
        # "Data names and types of shift register data are defined by this bundle."
        # "Initialize the shift-register data, here.\n(data names are defined by what you wire into the bundle function)"
        n134 = Bundle("Core"=w353, "Toolbar.Advance"=w350, "LoggerWatchDogQueue"=w348, "LogFile"=w349) -> (w355:T9)  [unwired: 1 in]
        n135 = call <vilib>:"Add State(s) to Queue__JKI_lib_State_Machine.vi"("State(s) in (\"\")"=w357) -> ("States Out"=w356:string)  [unwired: 14 in]
      }
      frame "Data: Initialize References" {
        n136 = control-ref of="Toolbar.Open BD"() -> (w361:refnum<vi>)
        n137 = control-ref of="Toolbar.Open FP"() -> (w362:refnum<vi>)
        n138 = Build Array(w361, w362) -> (w360:refnum<vi>[])
        n139 = Bundle By Name(cluster=w366, "Toolbar.Advance"=w360) -> (w363:T9)
      }
      frame "Data: Cleanup" {
        # "Cleanup any data and references, here.\n(this is called automatically, by the Macro: Exit)"
        n140 = Unbundle By Name(w371) -> ("Core.Current VI Reference"=w374:refnum<vi>)
        n141 = Close Reference(reference=w374, error in (no error)=w373) -> (error out=w372:errorcluster)
        n142 = call <vilib>:"Add State(s) to Queue__JKI_lib_State_Machine.vi"("State(s) in (\"\")"=w376) -> ("States Out"=w375:string)  [unwired: 14 in]
      }
      frame "---------- UI ----------" {
        # "Do not put any code in this frame.\n(It is a separator no-op. You can make a copy of this frame to create a new UI frame)"
        n143 = call <vilib>:"Add State(s) to Queue__JKI_lib_State_Machine.vi"("State(s) in (\"\")"=w383) -> ("States Out"=w382:string)  [unwired: 14 in]
      }
      frame "UI: Initialize" {
        # "Initialize the User Interface, here.\n(this is called automatically, by the Macro: Init)"
        n144 = Unbundle By Name(w387) -> ("Toolbar.Advance"=w386:refnum<vi>[])
        n145 = disable-structure shown="Disabled" {
          disable-tunnel: w386 -> [w393 _]
          frame Disabled {
            n146 = for {
              tunnel: w393 -> [w395] mode=indexing
              n147 = property class="Bool"(reference=w395, "Visible"=FALSE) -> ()  [unwired: 1 in, 2 out]
            }
          }
          frame Enabled {
          }
        }
        n148 = local write "Filter Peroid Logs"(TRUE ("Filter Peroid Logs")) -> ()
        n149 = call <vilib>:"Add State(s) to Queue__JKI_lib_State_Machine.vi"("State(s) in (\"\")"=w392) -> ("States Out"=w391:string)  [unwired: 14 in]
      }
      frame "UI: Cursor Set" {
        # "Argument"
        # "Set and Unset Cursor Busy.\n(Usage: \"UI: Cursor Set >> Busy|Idle\")"
        n150 = case shown="\"Idle\", Default" w399 {
          tunnel: w401 -> [w406 w408]
          tunnel: [w405 w407] -> w400
          frame "Idle", Default {
            n151 = call <vilib>:"Unset Busy.vi"("error in (no error)"=w406) -> ("error out"=w405:errorcluster)  [unwired: 10 in]
          }
          frame "Busy" {
            n152 = call <vilib>:"Set Busy.vi"("error in (no error)"=w408) -> ("error out"=w407:errorcluster)  [unwired: 9 in, 1 out]
          }
        }
        n153 = call <vilib>:"Add State(s) to Queue__JKI_lib_State_Machine.vi"("State(s) in (\"\")"=w404) -> ("States Out"=w403:string)  [unwired: 14 in]
      }
      frame "UI: Front Panel State" {
        # "Argument"
        # "Set Front Panel Open or Closed\n(Usage: \"UI: Front Panel State >> Open|Close\")"
        n154 = Unbundle By Name(w414) -> ("Core.Current VI Reference"=w413:refnum<vi>)
        n155 = case shown="\"Minimize\", \"Minimized\"" w412 {
          tunnel: w416 -> [w424 w439 w450 w463 w476]
          tunnel: [w426 w440 w452 w465 w478] -> w415
          tunnel: w413 -> [w425 w437 w451 w464 w477]
          frame "Open", "Standard", Default {
            w419 = T5."Standard" ("State")
            n156 = property class="VI"(reference=w425, error in=w424) -> (reference out=w422:refnum<vi>, error out=w423:errorcluster, "FP.State"=w421:T5)
            n157 = Not Equal?(x=w421, y=w419) -> (x != y?=w420:bool)
            n158 = case shown="True" w420 {
              tunnel: [w430 w432] -> w426
              tunnel: w423 -> [w429 w432]
              tunnel: w422 -> [w428 _]
              tunnel: w419 -> [w427 _]
              frame True {
                n159 = invoke class="VI" method="FP.Open"(reference=w428, error in=w429, "Activate"=TRUE, "State"=w427) -> (error out=w430:errorcluster)  [unwired: 1 in, 4 out]
              }
              frame False {
              }
            }
          }
          frame "Close", "Closed" {
            n160 = property class="VI"(reference=w437, error in=w439) -> (reference out=w436:refnum<vi>, error out=w438:errorcluster, "FP.State"=w434:T5)
            n161 = Not Equal?(x=w434, y=T5."Closed" ("Front Panel Window:State")) -> (x != y?=w433:bool)
            n162 = case shown="True" w433 {
              tunnel: [w441 w444] -> w440
              tunnel: w438 -> [w441 w443]
              tunnel: w436 -> [_ w442]
              frame False {
              }
              frame True {
                n163 = invoke class="VI" method="FP.Close"(reference=w442, error in=w443) -> (error out=w444:errorcluster)  [unwired: 1 in, 2 out]
              }
            }
          }
          frame "Hidden", "Hide" {
            w445 = T5."Hidden" ("State")
            n164 = property class="VI"(reference=w451, error in=w450) -> (reference out=w448:refnum<vi>, error out=w449:errorcluster, "FP.State"=w447:T5)
            n165 = Not Equal?(x=w447, y=w445) -> (x != y?=w446:bool)
            n166 = case shown="True" w446 {
              tunnel: [w456 w457] -> w452
              tunnel: w449 -> [w455 w457]
              tunnel: w448 -> [w454 _]
              tunnel: w445 -> [w453 _]
              frame True {
                n167 = invoke class="VI" method="FP.Open"(reference=w454, error in=w455, "State"=w453) -> (error out=w456:errorcluster)  [unwired: 2 in, 4 out]
              }
              frame False {
              }
            }
          }
          frame "Minimize", "Minimized" {
            w458 = T5."Minimized" ("State")
            n168 = property class="VI"(reference=w464, error in=w463) -> (reference out=w461:refnum<vi>, error out=w462:errorcluster, "FP.State"=w460:T5)
            n169 = Not Equal?(x=w460, y=w458) -> (x != y?=w459:bool)
            n170 = case shown="True" w459 {
              tunnel: [w469 w470] -> w465
              tunnel: w462 -> [w468 w470]
              tunnel: w461 -> [w467 _]
              tunnel: w458 -> [w466 _]
              frame True {
                n171 = invoke class="VI" method="FP.Open"(reference=w467, error in=w468, "State"=w466) -> (error out=w469:errorcluster)  [unwired: 2 in, 4 out]
              }
              frame False {
              }
            }
          }
          frame "Maximize", "Maximized" {
            w471 = T5."Maximized" ("State")
            n172 = property class="VI"(reference=w477, error in=w476) -> (reference out=w474:refnum<vi>, error out=w475:errorcluster, "FP.State"=w473:T5)
            n173 = Not Equal?(x=w473, y=w471) -> (x != y?=w472:bool)
            n174 = case shown="True" w472 {
              tunnel: [w482 w483] -> w478
              tunnel: w475 -> [w481 w483]
              tunnel: w474 -> [w480 _]
              tunnel: w471 -> [w479 _]
              frame True {
                n175 = invoke class="VI" method="FP.Open"(reference=w480, error in=w481, "State"=w479) -> (error out=w482:errorcluster)  [unwired: 2 in, 4 out]
              }
              frame False {
              }
            }
          }
        }
        n176 = call <vilib>:"Add State(s) to Queue__JKI_lib_State_Machine.vi"("State(s) in (\"\")"=w418) -> ("States Out"=w417:string)  [unwired: 14 in]
      }
      frame "UI: Refresh CSM List" {
        n177 = property on="CSM" class="CmbBox"() -> ("Value"=w488:string)  [unwired: 2 in, 2 out]
        n178 = call "CSM - List Modules.vi"() -> ("error out"=w485:errorcluster, "Module Names"=w490:string[])  [unwired: 10 in]
        n179 = Search 1D Array(1D array=w490, element=w488) -> (index of element=w486:i32)  [unwired: 1 in]
        n180 = Greater Or Equal To 0?(x=w486) -> (x >= 0?=w487:bool)
        n181 = Index Array(array=w490) -> (element=w489:string)  [unwired: 1 in]
        n182 = Select(t=w488, s=w487, f=w489) -> (s? t:f=w491:string)
        n183 = property on="CSM" class="CmbBox"("Strings[]"=w490, "Value"=w491) -> ()  [unwired: 2 in, 2 out]
        n184 = call <vilib>:"Simple Error Handler.vi"("error in (no error)"=w485) -> ()  [unwired: 4 in, 5 out]
      }
      frame "UI: Update Broadcast Registry" {
        n185 = call "CSM - List Mapping Relationships in Broadcast Registry.vi"() -> ("Mapping Relationships"=w498:T12)  [unwired: 10 in, 1 out]
        n186 = for {
          tunnel: w498 -> [w512] mode=indexing
          tunnel: [w505] -> w499 mode=indexing
          n187 = Unbundle(w512) -> (w511:string, "Name"=w510:string, "Target CSM"=w509:string, "Target State"=w508:string, "Register Type"=w507:T11)
          n188 = Format Into String(w507) -> (resulting string=w506:string)  [unwired: 3 in, 1 out]
          n189 = Build Array(w511, w510, w509, w508, w506) -> (w505:string[])
        }
        "Broadcast Registry" <- w499
      }
      frame "UI: Update Toolbar" {
        w521 = i16 2 ("x")
        n190 = control-ref of="Record.Start"() -> (w529:refnum<vi>)
        n191 = control-ref of="Record.Stop"() -> (w528:refnum<vi>)
        n192 = Unbundle By Name(w527) -> ("Core.Current VI Reference"=w518:refnum<vi>, "LogFile"=w515:path, "LoggerWatchDogQueue"=w526:refnum<queue>)
        n193 = Not A Number/Path/Refnum?(number/path/refnum=w526) -> (NaN/Path/Refnum?=w519:bool)
        n194 = Not(x=w519) -> (.not. x?=w520:bool)
        n195 = Boolean To (0,1)(Boolean=w520) -> (0, 1=w525:i16)
        n196 = Boolean To (0,1)(Boolean=w519) -> (0, 1=w524:i16)
        n197 = Multiply(x=w521, y=w524) -> (x*y=w522:i16)
        n198 = Multiply(x=w521, y=w525) -> (x*y=w523:i16)
        n199 = Empty String/Path?(string/path=w515) -> (empty?=w514:bool)
        n200 = property class="Bool"(reference=w529, "DisabledEnum"=w523) -> ()  [unwired: 1 in, 2 out]
        n201 = property class="Bool"(reference=w528, "DisabledEnum"=w522) -> ()  [unwired: 1 in, 2 out]
        n202 = case shown="True" w514 {
          tunnel: "Running Log Viewer (CSM)" ("Front Panel Window:Title") -> [w538 w539]
          tunnel: [w537 w539] -> w516
          tunnel: w515 -> [w534 _]
          frame False {
            n203 = Path To String(path=w534) -> (string=w535:string)
            n204 = Concatenate Strings(w538, " - " ("string"), w535) -> (w537:string)
          }
          frame True {
          }
        }
        n205 = property class="VI"(reference=w518, "Front Panel.Title"=w516) -> ()  [unwired: 1 in, 2 out]
      }
      frame "UI: Resize Tab Content" {
        w548 = u32 16 ("y")
        w544 = 8 ("Position:Left")
        n206 = control-ref of="Tab"() -> (w552:refnum<vi>)
        n207 = invoke class="TabCtl (strict)" method="FitControlToPane"(reference=w552) -> (reference out=w541:refnum<vi>)  [unwired: 2 in, 2 out]
        n208 = property class="TabCtl (strict)"(reference=w541) -> ("PaneHeight"=w550:u32, "PaneWidth"=w549:u32, "TabHeight"=w543:u32)  [unwired: 1 in, 2 out]
        n209 = control-ref of="Broadcast Registry"() -> (w547:refnum<vi>)
        n210 = control-ref of="Error History"() -> (w551:refnum<vi>)
        n211 = Subtract(x=w549, y=w548) -> (x-y=w545:u32)
        n212 = Subtract(x=w550, y=w548) -> (x-y=w546:u32)
        n213 = Add(x=w544, y=w543) -> (x+y=w542:u32)
        n214 = property class="Str"(reference=w551, "Left"=w544, "Top"=w542, "Height"=w546, "Width"=w545) -> ()  [unwired: 1 in, 2 out]
        n215 = property class="Tbl (strict)"(reference=w547, "Left"=w544, "Top"=w542, "Height"=w546, "Width"=w545) -> ()  [unwired: 1 in, 2 out]
      }
      frame "---------- Macro ----------" {
        # "Do not put any code in this frame.\n(It is a separator no-op. You can make a copy of this frame to create a new Macro frame)"
        n216 = call <vilib>:"Add State(s) to Queue__JKI_lib_State_Machine.vi"("State(s) in (\"\")"=w564) -> ("States Out"=w563:string)  [unwired: 14 in]
      }
      frame "Macro: Initialize" {
        w568 = "Data: Initialize\nData: Initialize References\nInitialize Core Data\nUI: Initialize\nUI: Front Panel State >> Open\nUI: Resize Tab Content\nUI: Refresh CSM List\nUI: Update Broadcast Registry\nUI: Update Toolbar"  # Data: Initialize Data: Initialize References Initialize Core Data UI: Initialize UI: Front Panel State >> Open UI: Resize Tab Content UI: Refresh CSM List UI: Update Broadcast Registry UI: Update Toolbar
        # "Initialization Macro\n(This is called once, when the VI starts)"
        n217 = call <vilib>:"Add State(s) to Queue__JKI_lib_State_Machine.vi"("State(s) in Front (\"\")"=w568, "State(s) in (\"\")"=w572) -> ("States Out"=w571:string)  [unwired: 13 in]
      }
      frame "Macro: Exit" {
        # "Exit Macro\n(This is called once, when the VI exits)"
        n218 = Unbundle By Name(w582) -> ("Core.Close Panel on Exit?"=w581:bool)
        n219 = Select(t="UI: Front Panel State >> Close", s=w581, f="") -> (s? t:f=w578:string)
        n220 = call <vilib>:"Add State(s) to Queue__JKI_lib_State_Machine.vi"("State(s) in (\"\")"=w578, "State(s) at Back (\"\")"="Data: Cleanup\nExit") -> ("States Out"=w576:string)  [unwired: 13 in]
        n221 = call <vilib>:"Add State(s) to Queue__JKI_lib_State_Machine.vi"("State(s) in Front (\"\")"=w576, "State(s) in (\"\")"=w585) -> ("States Out"=w584:string)  [unwired: 13 in]
      }
    }
  }
  n222 = call "CSM - Destroy Global Log Event.vi"("Error In"=w5, "CSM Global Log Event"=w11) -> ("error out"=w4:errorcluster)  [unwired: 9 in]
  n223 = invoke class="VI" method="FP.Close"(error in=w4) -> (error out=w13:errorcluster)  [unwired: 2 in, 2 out]
  n224 = call <vilib>:"Clear Errors.vi"("error in (no error)"=w13) -> ()  [unwired: 5 in, 2 out]
